vi "FullAdder.vi"(2 "Cin":bool, 3 "B":bool, 4 "A":bool) -> (0 "Cout":bool, 1 "S":bool)   [LabVIEW 2015]
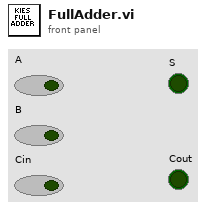
[diagram p1: front panel]
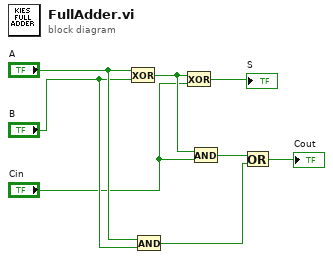
[diagram p0: block diagram]
diagram:
  n1 = Exclusive Or(1:"B", 2:"A") -> (0:w6:bool)
  n2 = And(x="A", y="B") -> (x .and. y?=w3:bool)
  n3 = Exclusive Or(1:"Cin", 2:w6) -> (0:→"S":bool)
  n4 = And(x=w6, y="Cin") -> (x .and. y?=w4:bool)
  n5 = Or(x=w4, y=w3) -> (x .or. y?=→"Cout":bool)
